vi "PCO_SetIntensifiedLoopCount.vi"(8 "error in (no error)":errorcluster {"code" format="%x"}, 10 "wIntensifiedLoopCount":u16, 11 "ph":u64) -> (0 "error out":errorcluster {"code" format="%x"}, 2 "ErrorMessage":i32 format="%x", 3 "ph out":u64)   [LabVIEW 2019, in "SDK.lvlib" / "SpecialCommandsDicam.lvlib"]
doc: "SC2_SDK_FUNC int WINAPI PCO_SetIntensifiedLoopCount(HANDLE hCam, WORD wIntensifiedLoopCount, WORD wReserved);"
uses:
  SpecialCommandsDicam.lvlib
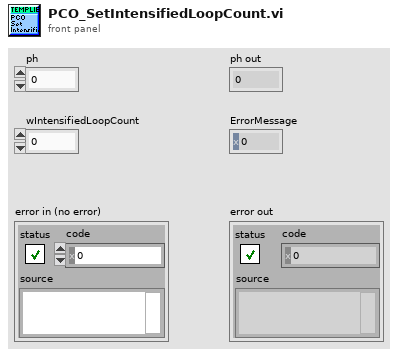
[diagram p1: front panel]
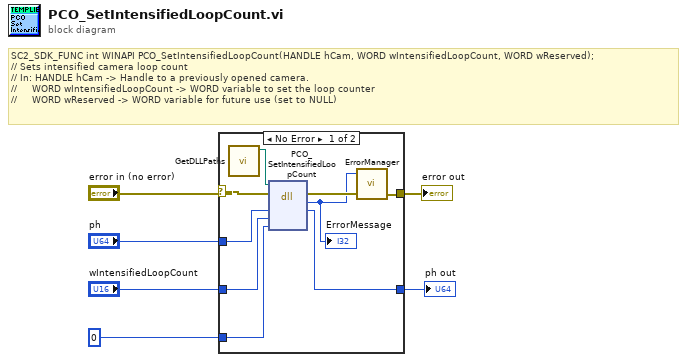
[diagram p0: block diagram]
diagram:
  # "SC2_SDK_FUNC int WINAPI PCO_SetIntensifiedLoopCount(HANDLE hCam, WORD wIntensifiedLoopCount, WORD wReserved);\n// Sets intensified camera loop count\n// In: HANDLE hCam -> Handle to a previously opened camera.\n//     WORD wIntensifiedLoopCount -> WORD variable to set the loop counter\n//     WORD wReserved -> WORD variable for future use (set to NULL)"
  n1 = case shown="No Error" "error in (no error)" {
    selector: "error in (no error)" -> [w11 w17]
    tunnel: "ph" -> [w15 w16]
    tunnel: [w14 w16] -> w5
    tunnel: "wIntensifiedLoopCount" -> [w13 _]
    tunnel: [w10 w17] -> w3
    tunnel: u16 0 ("wReserved") -> [w12 _]
    frame No Error {
      n2 = call "GetDLLPaths.vi"() -> ("SC2_Cam_Path"=w7:path)  [unwired: 8 in, 3 out]
      n3 = dll-call lib="?" fn="PCO_SetIntensifiedLoopCount"(path in=w7, error in=w11, "ph"=w15, "wIntensifiedLoopCount"=w13, "wReserved"=w12) -> (error out=w9:errorcluster, "return type"=w8:i32, "ph"=w14:u64)  [unwired: 3 in, 1 out]
      "ErrorMessage" <- w8
      n4 = call "ErrorManager.vi"("error in (no error)"=w9, "error code"=w8) -> ("error out"=w10:errorcluster)  [unwired: 2 in, 1 out]
    }
    frame Error {
    }
  }
  "ph out" <- w5
  "error out" <- w3
